vi "TDMS File Read.vi"(4 "count (-1: all)":i64=-1, 6 "offset (0)":i64, 7 "Use input reference (F)":bool, 8 "Error In":errorcluster, 9 "Channel to load":enum16{"Red", "Green", "Both"}(ring)=enum."Both", 10 "tdms file ref":refnum<k34>, 11 "File Path":path) -> (0 "Error Out":errorcluster, 1 "Single channel data":dbl[](array[numeric]), 2 "tdms file out":refnum<k34>, 3 "Data":waveform(dbl)[](array[waveform]), 5 "Double channel data":dbl[][](array[numeric]))   [LabVIEW 2020]
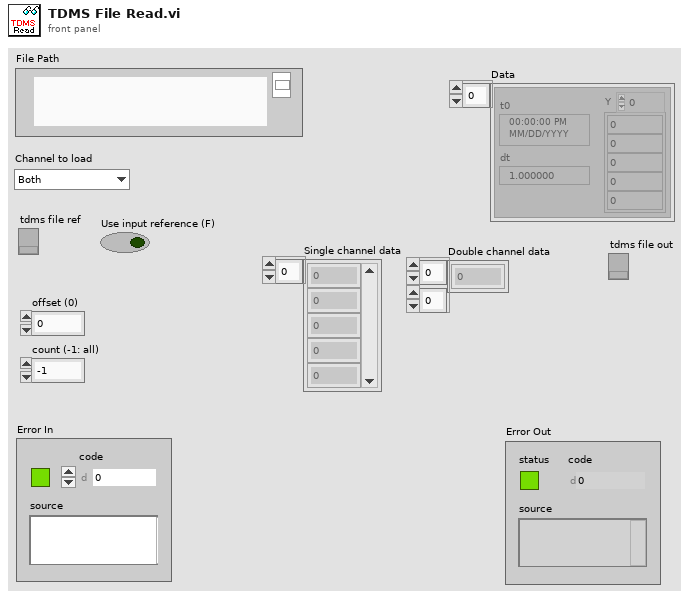
[diagram p1: front panel]
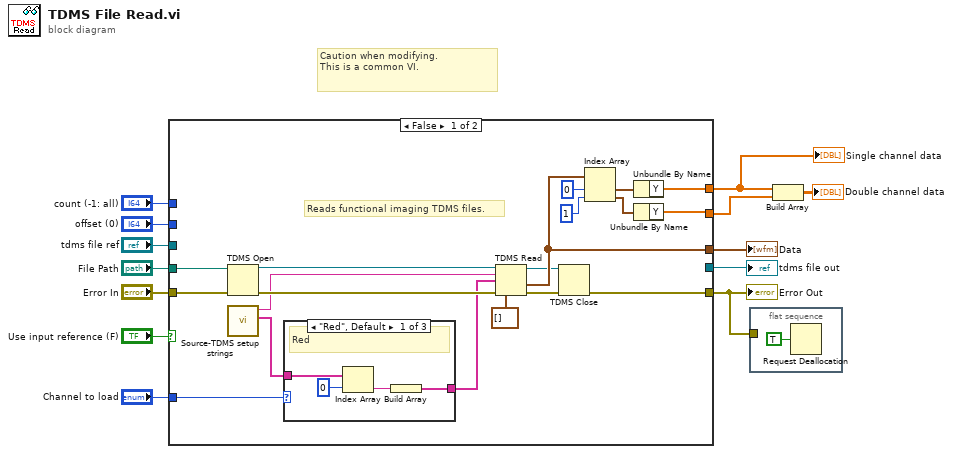
[diagram p0: block diagram]
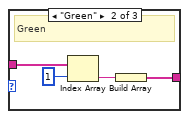
[diagram p2: hidden frame]
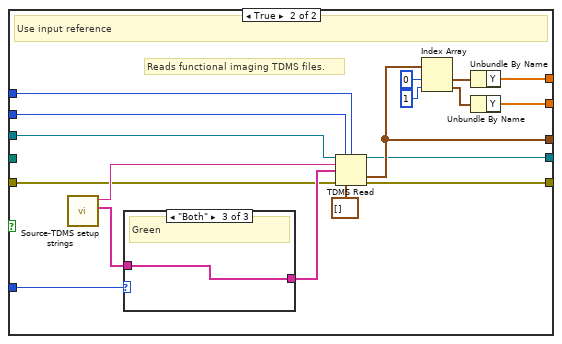
[diagram p4: hidden frame]
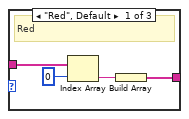
[diagram p5: hidden frame]
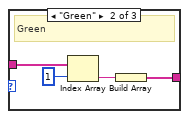
[diagram p6: hidden frame]
diagram:
  # "Caution when modifying.\nThis is a common VI."
  n1 = case shown="False" "Use input reference (F)" {
    tunnel: "File Path" -> [w31 _]
    tunnel: "Error In" -> [w27 w47]
    tunnel: [w25 w48] -> w6
    tunnel: "Channel to load" -> [w24 w57]
    tunnel: [w19 w52] -> w10
    tunnel: [w18 w51] -> w3
    tunnel: "tdms file ref" -> [_ w50]
    tunnel: [_ w49] -> w7
    tunnel: "offset (0)" -> [_ w46]
    tunnel: "count (-1: all)" -> [_ w45]
    tunnel: [w14 w42] -> w2
    frame False {
      # "Reads functional imaging TDMS files."
      n2 = TDMS Open(8:w27, 11:w31) -> (0:w29:errorcluster, 3:w30:refnum<k34>)  [unwired: 5 in]
      n3 = call "Source-TDMS setup strings.vi"() -> ("Functional imaging TDMS channel names array"=w23:string[], "TDMS group name"=w26:string)  [unwired: 10 in]
      n4 = case shown="\"Red\", Default" w24 {
        tunnel: [w34 w38 w41] -> w22
        tunnel: w23 -> [w33 w37 w41]
        frame "Red", Default {
          # "Red"
          n5 = Index Array(array=w33, index=0) -> (element=w35:string)
          n6 = Build Array(w35) -> (w34:string[])
        }
        frame "Green" {
          # "Green"
          n7 = Index Array(array=w37, index=1) -> (element=w39:string)
          n8 = Build Array(w39) -> (w38:string[])
        }
        frame "Both" {
          # "Green"
        }
      }
      n9 = TDMS Read(0:w30, 5:w26, 7:w22, 11:w29, 12:waveform(dbl)[] [] ("data type")) -> (4:w17:refnum<k34>, 10:w19:waveform(dbl)[], 15:w28:errorcluster)  [unwired: 3 in, 3 out]
      n10 = TDMS Close(8:w28, 11:w17) -> (0:w25:errorcluster)  [unwired: 1 out]
      n11 = Index Array(array=w19, index #1=0 ("index"), index #2=1 ("index")) -> (element #1=w21:waveform(dbl), element #2=w15:waveform(dbl))
      n12 = Unbundle By Name ("Get Waveform Components")(w21) -> ("Y"=w18:dbl[])
      n13 = Unbundle By Name ("Get Waveform Components")(w15) -> ("Y"=w14:dbl[])
    }
    frame True {
      # "Reads functional imaging TDMS files."
      # "Use input reference"
      n14 = call "Source-TDMS setup strings.vi"() -> ("Functional imaging TDMS channel names array"=w56:string[], "TDMS group name"=w58:string)  [unwired: 10 in]
      n15 = case shown="\"Both\"" w57 {
        tunnel: [w61 w65 w68] -> w55
        tunnel: w56 -> [w60 w64 w68]
        frame "Red", Default {
          # "Red"
          n16 = Index Array(array=w60, index=0) -> (element=w62:string)
          n17 = Build Array(w62) -> (w61:string[])
        }
        frame "Green" {
          # "Green"
          n18 = Index Array(array=w64, index=1) -> (element=w66:string)
          n19 = Build Array(w66) -> (w65:string[])
        }
        frame "Both" {
          # "Green"
        }
      }
      n20 = TDMS Read(0:w50, 1:w46, 2:w45, 5:w58, 7:w55, 11:w47, 12:waveform(dbl)[] [] ("data type")) -> (4:w49:refnum<k34>, 10:w52:waveform(dbl)[], 15:w48:errorcluster)  [unwired: 1 in, 3 out]
      n21 = Index Array(array=w52, index #1=0 ("index"), index #2=1 ("index")) -> (element #1=w54:waveform(dbl), element #2=w43:waveform(dbl))
      n22 = Unbundle By Name ("Get Waveform Components")(w54) -> ("Y"=w51:dbl[])
      n23 = Unbundle By Name ("Get Waveform Components")(w43) -> ("Y"=w42:dbl[])
    }
  }
  "Error Out" <- w6
  "Data" <- w10
  "Single channel data" <- w3
  "tdms file out" <- w7
  n24 = flat-sequence {
    tunnel: w6 -> [_]
    frame #0 {
      n25 = Request Deallocation(TRUE ("flag")) -> ()
    }
  }
  n26 = Build Array(w3, w2) -> (→"Double channel data":dbl[][])
